vi "TestCycleRamp1.vi"(11 "TestCycleParameters":T1={"TAmb"=20.0, "HeaterTestTemp"=-80.0, "HeaterTestDwell(min)"=30, "HeaterTestDuration"=15, "MinOpTemp"=-50.0, "MinOpDwell(min)"=30, "TestHeatingRate (deg/min)"=0.4, "SurviveCycleParameters"={"MinSurviveTemp"=-130.0, "MinSurvive Dwell(min)"=60, "MaxSurviveTemp"=50.0, "MaxSurviveDwell(min)"=30, "ControlInput"=0, "ColdStandOff"=-50.0, "HotStandoff"=0.0, "SteadyPWM"=20, "MaxCoolingRate (deg/min)"=3.75, "MaxHeatingRate (deg/min)"=2.5}, "CycleType"=0, "MaxOpTemp"=40.0, "MaxOpDwell(min)"=30} {"CycleType" items=["Survival", "Operational"]; "SurviveCycleParameters"."SteadyPWM" min=0 max=100 step=1; "SurviveCycleParameters"."ControlInput" items=["3A", "3B", "3C", "3D", "4A", "4B", "4C", "4D"]}) -> (3 "Profile":cluster{dbl[], dbl[]}(graph)={[0.0, 40.0, 100.0, 120.0, 150.0, 165.0, 177.0, 207.0, 432.0, 462.0], [20.0, -130.0, -130.0, -80.0, -80.0, -80.0, -50.0, -50.0, 40.0, 40.0]})   [LabVIEW 2024]
uses:
  controls/TestCycleParams.ctl
  controls/SurviveCycleParams.ctl
  controls/ControlInput.ctl
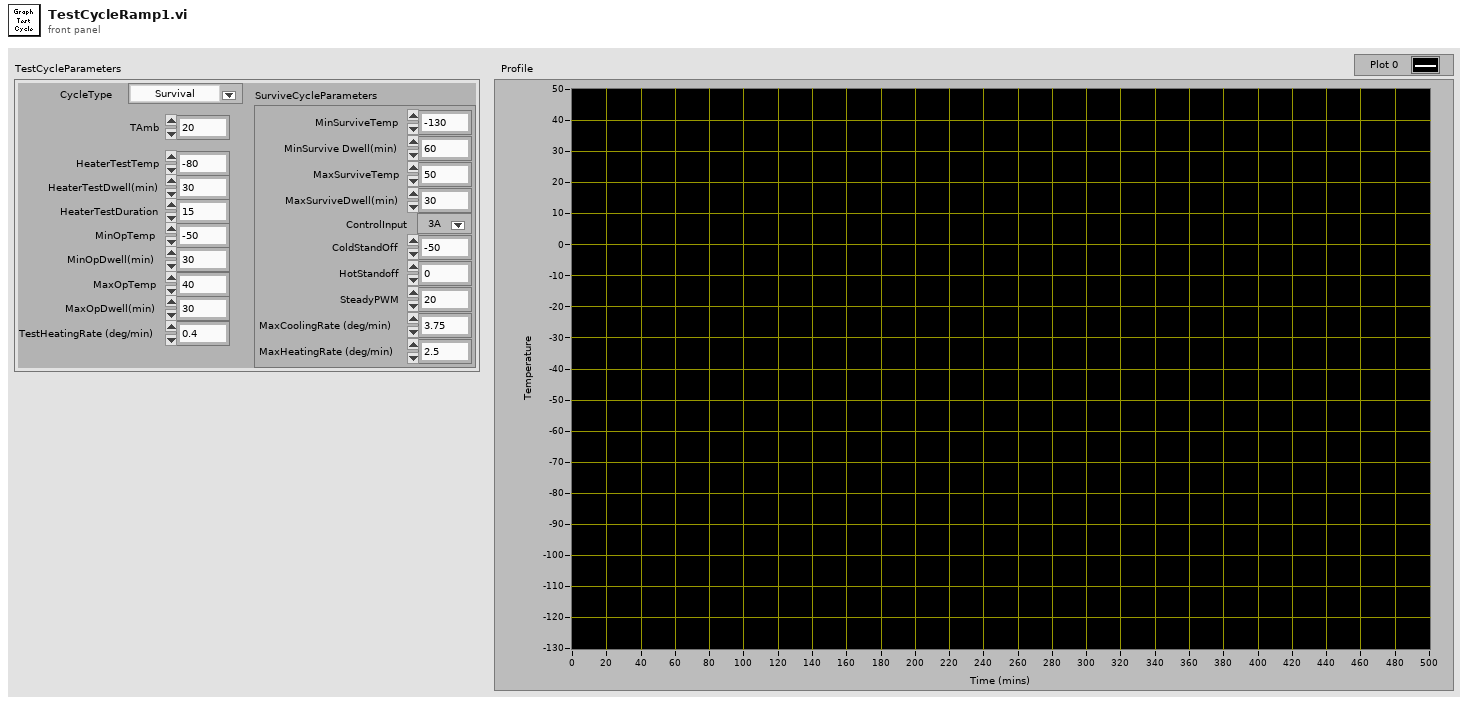
[diagram p1: front panel]
types:
  T1 = typedef "TestCycleParams.ctl" = cluster{"TAmb":dbl, "HeaterTestTemp":dbl, "HeaterTestDwell(min)":i32, "HeaterTestDuration":i32, "MinOpTemp":dbl, "MinOpDwell(min)":i32, "TestHeatingRate (deg/min)":dbl, "SurviveCycleParameters":T2, "CycleType":u16, "MaxOpTemp":dbl, "MaxOpDwell(min)":i32}
  T2 = typedef "SurviveCycleParams.ctl" = cluster{"MinSurviveTemp":dbl, "MinSurvive Dwell(min)":i32, "MaxSurviveTemp":dbl, "MaxSurviveDwell(min)":i32, "ControlInput":T3, "ColdStandOff":dbl, "HotStandoff":dbl, "SteadyPWM":i32, "MaxCoolingRate (deg/min)":dbl, "MaxHeatingRate (deg/min)":dbl}
  T3 = typedef "ControlInput.ctl" = u16
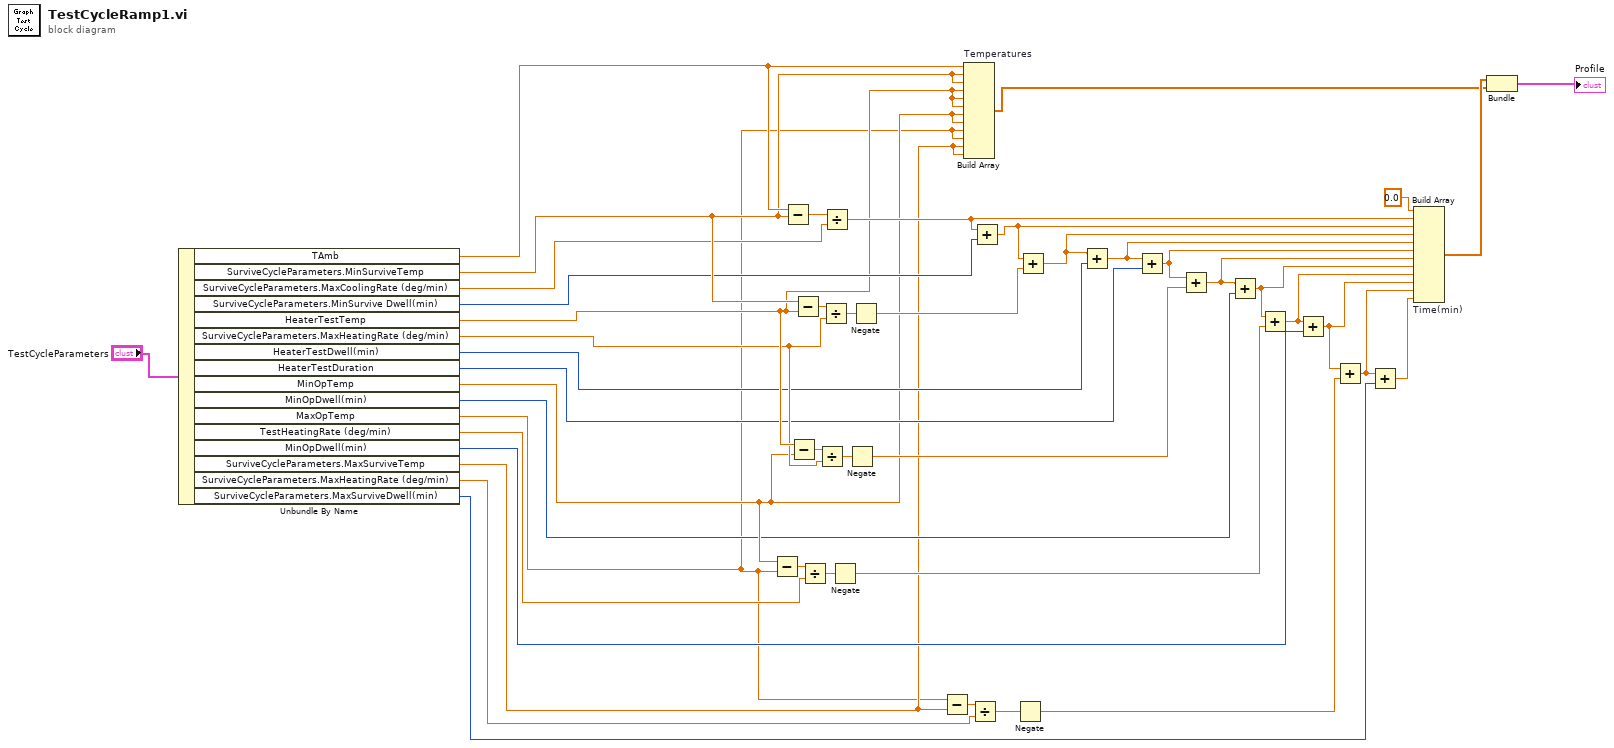
[diagram p0: block diagram]
diagram:
  n1 = Unbundle By Name("TestCycleParameters") -> ("TAmb"=w23:dbl, "SurviveCycleParameters.MinSurviveTemp"=w22:dbl, "SurviveCycleParameters.MaxCoolingRate (deg/min)"=w21:dbl, "SurviveCycleParameters.MinSurvive Dwell(min)"=w20:i32, "HeaterTestTemp"=w19:dbl, "SurviveCycleParameters.MaxHeatingRate (deg/min)"=w18:dbl, "HeaterTestDwell(min)"=w17:i32, "HeaterTestDuration"=w16:i32, "MinOpTemp"=w15:dbl, "MinOpDwell(min)"=w14:i32, "MaxOpTemp"=w2:dbl, "TestHeatingRate (deg/min)"=w13:dbl, "MinOpDwell(min)"=w12:i32, "SurviveCycleParameters.MaxSurviveTemp"=w4:dbl, "SurviveCycleParameters.MaxHeatingRate (deg/min)"=w9:dbl, "SurviveCycleParameters.MaxSurviveDwell(min)"=w3:i32)
  n2 = Subtract(x=w15, y=w2) -> (x-y=w27:dbl)
  n3 = Subtract(x=w23, y=w22) -> (x-y=w44:dbl)
  n4 = Subtract(x=w19, y=w15) -> (x-y=w33:dbl)
  n5 = Subtract(x=w22, y=w19) -> (x-y=w39:dbl)
  n6 = Divide(x=w27, y=w13) -> (x/y=w28:dbl)
  n7 = Divide(x=w33, y=w18) -> (x/y=w32:dbl)
  n8 = Divide(x=w39, y=w18) -> (x/y=w38:dbl)
  n9 = Divide(x=w44, y=w21) -> (x/y=w43:dbl)
  n10 = Negate(x=w28) -> (-x=w10:dbl)
  n11 = Negate(x=w32) -> (-x=w30:dbl)
  n12 = Negate(x=w38) -> (-x=w36:dbl)
  n13 = Subtract(x=w2, y=w4) -> (x-y=w11:dbl)
  n14 = Build Array "Temperatures"(w23, w22, w22, w19, w19, w19, w15, w15, w2, w2, w4, w4) -> (w41:dbl[])
  n15 = Divide(x=w11, y=w9) -> (x/y=w7:dbl)
  n16 = Add(x=w43, y=w20) -> (x+y=w37:dbl)
  n17 = Negate(x=w7) -> (-x=w1:dbl)
  n18 = Add(x=w37, y=w36) -> (x+y=w35:dbl)
  n19 = Add(x=w35, y=w17) -> (x+y=w34:dbl)
  n20 = Add(x=w34, y=w16) -> (x+y=w31:dbl)
  n21 = Add(x=w31, y=w30) -> (x+y=w29:dbl)
  n22 = Add(x=w29, y=w14) -> (x+y=w26:dbl)
  n23 = Add(x=w26, y=w10) -> (x+y=w25:dbl)
  n24 = Add(x=w25, y=w12) -> (x+y=w8:dbl)
  n25 = Add(x=w8, y=w1) -> (x+y=w6:dbl)
  n26 = Add(x=w6, y=w3) -> (x+y=w5:dbl)
  n27 = Build Array "Time(min)"(0.0, w43, w37, w35, w34, w31, w29, w26, w25, w8, w6, w5) -> (w42:dbl[])
  n28 = Bundle(w42, w41) -> (→"Profile":cluster{dbl[], dbl[]})  [unwired: 1 in]
